vi "FinishAcquisition.vi"(7 "Application Data":T4, 8 "error in (no error)":errorcluster, 11 "Acq Thread Data":T1) -> (0 "error out":errorcluster, 3 "Acq Thread Data out":T1)   [LabVIEW 2019]
uses:
  Typedefs/Acquisition Thread/#cluster_AcqThreadData.ctl
  <vilib>/MagicBox/Device/Arduino/Arduino.lvclass
  <vilib>/MagicBox/Peripherals/POX/POX.lvclass
  Typedefs/Acquisition Thread/#enum_AcqThreadState.ctl
  Typedefs/#cluster_GUIRefs.ctl
  Typedefs/#cluster_ApplicationData.ctl
  Typedefs/Acquisition Thread/#cluster_AcqQueueData.ctl
  Typedefs/Acquisition Thread/#enum_AcquisitionTask.ctl
  Typedefs/Saving Thread/#cluster_SavingQueueData.ctl
  Typedefs/Saving Thread/#enum_SavingTask.ctl
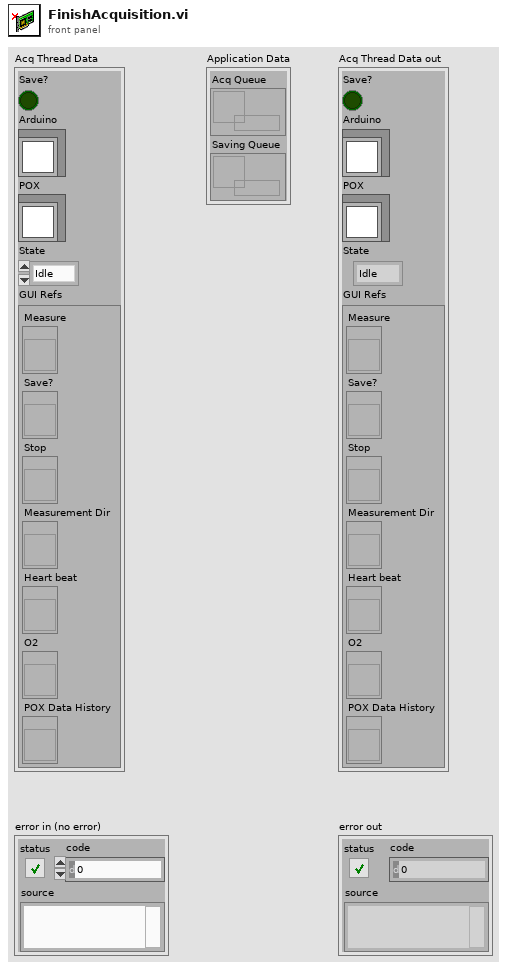
[diagram p1: front panel]
types:
  T1 = typedef "#cluster_AcqThreadData.ctl" = cluster{"Save?":bool, "Arduino":refnum<class "Arduino.lvclass">, "POX":refnum<class "POX.lvclass">, "State":T2, "GUI Refs":T3}
  T2 = typedef "#enum_AcqThreadState.ctl" = enum16{"Idle", "Operate", "Error"}
  T3 = typedef "#cluster_GUIRefs.ctl" = cluster{"Measure":refnum<vi>, "Save?":refnum<vi>, "Stop":refnum<vi>, "Measurement Dir":refnum<vi>, "Heart beat":refnum<vi>, "O2":refnum<vi>, "POX Data History":refnum<vi>}
  T4 = typedef "#cluster_ApplicationData.ctl" = cluster{"Acq Queue":refnum<queue>, "Saving Queue":refnum<queue>}
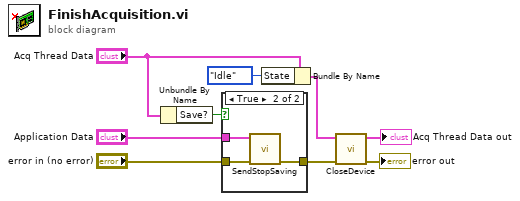
[diagram p0: block diagram]
diagram:
  n1 = Unbundle By Name("Acq Thread Data") -> ("Save?"=w6:bool)
  n2 = case shown="True" w6 {
    tunnel: "error in (no error)" -> [w10 w13]
    tunnel: [w10 w12] -> w4
    tunnel: "Application Data" -> [_ w11]
    frame False {
    }
    frame True {
      n3 = call "SendStopSaving.vi"("error in (no error)"=w13, "Application Data"=w11) -> ("error out"=w12:errorcluster)  [unwired: 9 in]
    }
  }
  n4 = Bundle By Name(cluster="Acq Thread Data", "State"=#enum_AcqThreadState."Idle") -> (w8:T1)
  n5 = call "CloseDevice.vi"("error in (no error)"=w4, "Acq Thread Data in"=w8) -> ("error out"=→"error out":errorcluster, "Acq Thread Data out"=→"Acq Thread Data out":T1)  [unwired: 8 in]
